vi "SVFA FFT Spectrum (Complex).vi"   [LabVIEW 2017]
doc: "Computes the Fast Fourier Transform (FFT) spectrum of <B>scaled signal [EU]</B>. This VI returns FFT results as the complex form of the FFT spectrum. Wire data to the <B>scaled signal [EU]</B> input to determine the polymorphic instance to use or manually select the instance."
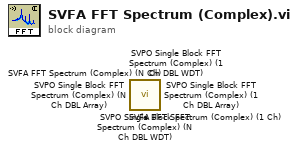
[diagram p0: block diagram]
diagram:
  n1 = call <vilib>:"SVPO Single Block FFT Spectrum (Complex) (N Ch DBL WDT).vi"() -> ()  [unwired: 19 in, 1 out]
  n2 = call <vilib>:"SVPO Single Block FFT Spectrum (Complex) (1 Ch DBL WDT).vi"() -> ()  [unwired: 19 in, 1 out]
  n3 = call <vilib>:"SVPO Single Block FFT Spectrum (Complex) (N Ch DBL Array).vi"() -> ()  [unwired: 19 in, 1 out]
  n4 = call <vilib>:"SVPO Single Block FFT Spectrum (Complex) (1 Ch DBL Array).vi"() -> ()  [unwired: 19 in, 1 out]
  n5 = call <vilib>:"SVFA FFT Spectrum (Complex) (N Ch).vi"() -> ()  [unwired: 16 in, 4 out]
  n6 = call <vilib>:"SVFA FFT Spectrum (Complex) (1 Ch).vi"() -> ()  [unwired: 16 in, 4 out]
